vi "Read Shutdown Event.vi"(11 "Controller Interface in":refnum<class "Controller Interface.lvclass">) -> (2 "Shutdown Event":refnum<user-event>, 3 "Controller Interface out":refnum<class "Controller Interface.lvclass">)   [LabVIEW 2019, in "Controller Interface.lvlib" / "Controller Interface.lvclass"]
uses:
  Controller Interface.lvclass
  Controller Interface.lvclass/Controller Interface.ctl
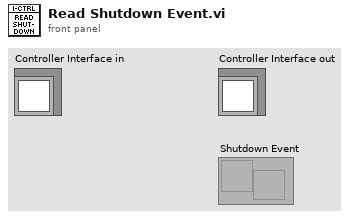
[diagram p1: front panel]
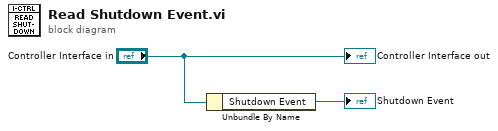
[diagram p0: block diagram]
diagram:
  n1 = Unbundle By Name("Controller Interface in") -> ("Shutdown Event"=→"Shutdown Event":refnum<user-event>)
  "Controller Interface out" <- "Controller Interface in"
